vi "UNIX_Time.vi"(8 "error in (no error)":errorcluster) -> (0 "error out":errorcluster, 3 "Unix time - UTC":u32)   [LabVIEW 2013]
doc: "Outputs the current UNIX time (converts from the 1904 epoch LabVIEW based time to the 1970 UNIX epoch time). In addition, this VI takes into account the current time zone (and daylight saving settings) you have on your computer to get the accurate UNIX time conversion."
uses:
  <vilib>/Utility/miscctls.llb/LVDateTimeRec.ctl
  kernel32.dll
panel:
  out "date time rec":T1
  out "In Daylight Savings?":bool
  out "Unix UTC":timestamp
  out "Sample UTC calc":u32
  out "Local time stamp":timestamp
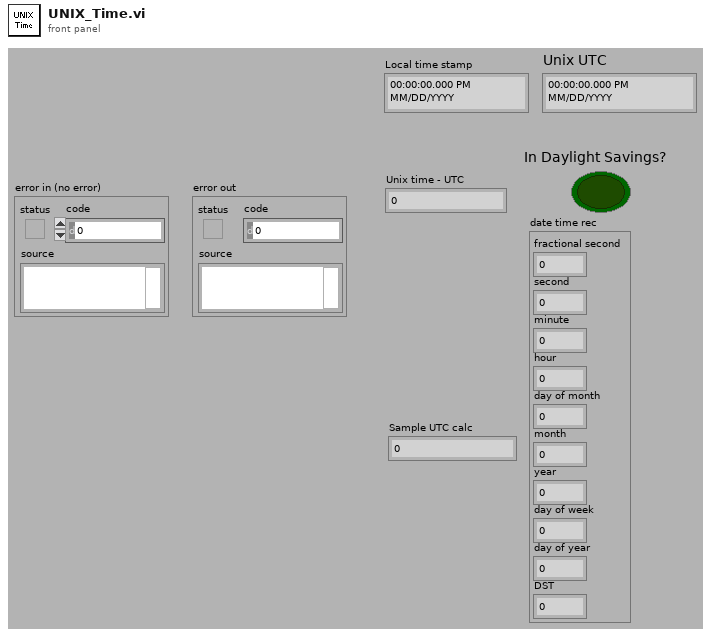
[diagram p1: front panel]
types:
  T1 = typedef "LVDateTimeRec.ctl" = cluster{"fractional second":dbl, "second":i32, "minute":i32, "hour":i32, "day of month":i32, "month":i32, "year":i32, "day of week":i32, "day of year":i32, "DST":i32}
  T2 = cluster{"[0]":u16, "[1]":u16, "[2]":u16, "[3]":u16, "[4]":u16, "[5]":u16, "[6]":u16, "[7]":u16, "[8]":u16, "[9]":u16, "[10]":u16, "[11]":u16, "[12]":u16, "[13]":u16, "[14]":u16, "[15]":u16, "[16]":u16, "[17]":u16, "[18]":u16, "[19]":u16, "[20]":u16, "[21]":u16, "[22]":u16, "[23]":u16, "[24]":u16, "[25]":u16, "[26]":u16, "[27]":u16, "[28]":u16, "[29]":u16, "[30]":u16, "[31]":u16, "[32]":u16, "[33]":u16, "[34]":u16, "[35]":u16, "[36]":u16, "[37]":u16, "[38]":u16, "[39]":u16, "[40]":u16, "[41]":u16, "[42]":u16, "[43]":u16, "[44]":u16, "[45]":u16, "[46]":u16, "[47]":u16, "[48]":u16, "[49]":u16, "[50]":u16, "[51]":u16, "[52]":u16, "[53]":u16, "[54]":u16, "[55]":u16, "[56]":u16, "[57]":u16, "[58]":u16, "[59]":u16, "[60]":u16, "[61]":u16, "[62]":u16, "[63]":u16, "[64]":u16, "[65]":u16, "[66]":u16, "[67]":u16, "[68]":u16, "[69]":u16, "[70]":u16, "[71]":u16, "[72]":u16, "[73]":u16, "[74]":u16, "[75]":u16, "[76]":u16, "[77]":u16, "[78]":u16, "[79]":u16, "[80]":u16, "[81]":u16, "[82]":u16, "[83]":u16, "[84]":u16, "[85]":u16}
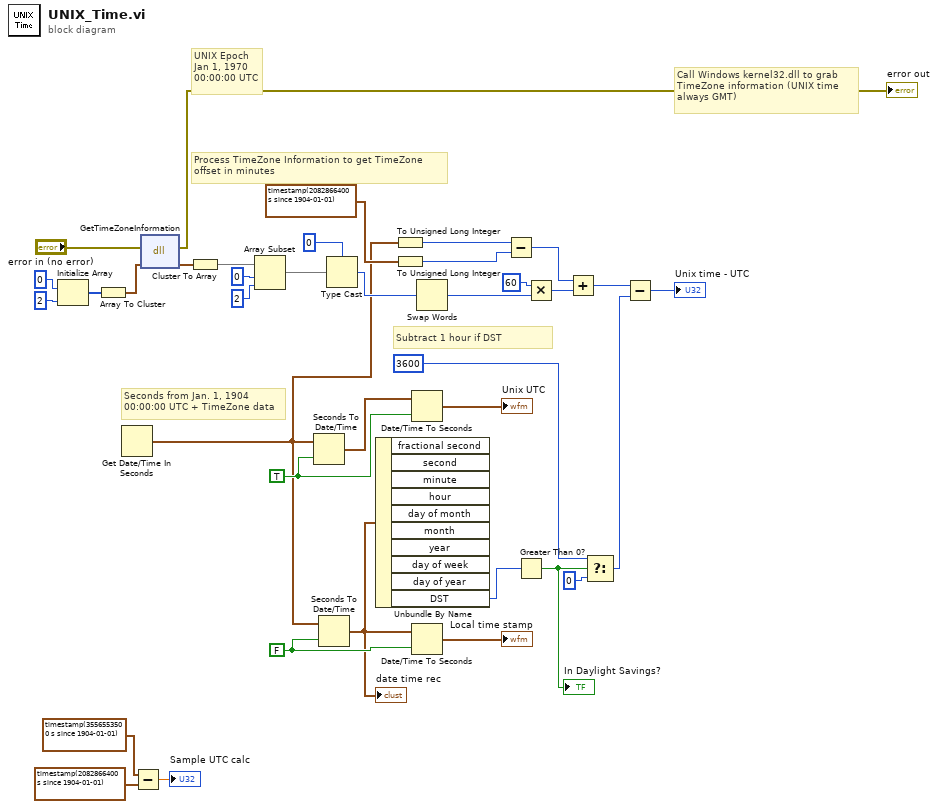
[diagram p0: block diagram]
diagram:
  w3 = TRUE ("to UTC (F)")
  w16 = FALSE ("to UTC (F)")
  # "Subtract 1 hour if DST"
  # "Seconds from Jan. 1, 1904\n00:00:00 UTC + TimeZone data"
  # "UNIX Epoch\nJan 1, 1970\n00:00:00 UTC"
  # "Process TimeZone Information to get TimeZone\noffset in minutes"
  # "Call Windows kernel32.dll to grab\nTimeZone information (UNIX time\nalways GMT)"
  n1 = Initialize Array(u16 0 ("element"), 2 ("dimension size")) -> (w34:u16[])
  n2 = Array To Cluster(array=w34) -> (cluster=w31:T2)
  n3 = Get Date/Time In Seconds() -> (seconds since 1Jan1904=w2:timestamp)
  n4 = Subtract(x=timestamp(3556553500 s since 1904-01-01), y=timestamp(2082866400 s since 1904-01-01)) -> (x-y=→"Sample UTC calc":dbl)
  n5 = dll-call lib="kernel32.dll" fn="GetTimeZoneInformation"(error in="error in (no error)", "lpTimeZoneInformation"=w31) -> (error out=→"error out":errorcluster, "lpTimeZoneInformation"=w30:T2)  [unwired: 2 in, 2 out]
  n6 = Cluster To Array(cluster=w30) -> (array=w29:u16[])
  n7 = Array Subset(array=w29, index=0, length=2) -> (w25:u16[])
  n8 = Seconds To Date/Time(time stamp (now)=w2, to UTC (F)=w3) -> (date time rec=w4:T1)
  n9 = Seconds To Date/Time(time stamp (now)=w2, to UTC (F)=w16) -> (date time rec=w15:T1)
  "date time rec" <- w15
  n10 = Type Cast(type=0, x=w25) -> (*(type *) &x=w24:i32)
  n11 = Unbundle By Name(w15) -> ("DST"=w12:i32)  [unwired: 9 out]
  n12 = To Unsigned Long Integer(number=w2) -> (unsigned 32bit integer=w36:u32)
  n13 = To Unsigned Long Integer(number=timestamp(2082866400 s since 1904-01-01)) -> (unsigned 32bit integer=w35:u32)
  n14 = Date/Time To Seconds(1:w3, 2:w4) -> (0:→"Unix UTC":timestamp)
  n15 = Date/Time To Seconds(1:w16, 2:w15) -> (0:→"Local time stamp":timestamp)
  n16 = Swap Words(1:w24) -> (0:w21:i32)
  n17 = Subtract(x=w36, y=w35) -> (x-y=w23:u32)
  n18 = Greater Than 0?(x=w12) -> (x > 0?=w11:bool)
  "In Daylight Savings?" <- w11
  n19 = Multiply(x=u32 60 ("y"), y=w21) -> (x*y=w22:u32)
  n20 = Add(x=w23, y=w22) -> (x+y=w7:u32)
  n21 = Select(t=u32 3600, s=w11, f=u32 0) -> (s? t:f=w6:u32)
  n22 = Subtract(x=w7, y=w6) -> (x-y=→"Unix time - UTC":u32)
